vi "Create.vi"(10 "Groups":string[](array[string])) -> (3 "GroupsValue out":refnum<class "GroupsValue.lvclass">)   [LabVIEW 2020, in "Vecto.lvlib" / "GroupsValue.lvclass"]
uses:
  GroupsValue.lvclass
  GroupsValue.lvclass/GroupsValue.ctl
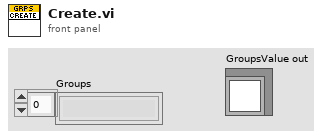
[diagram p1: front panel]
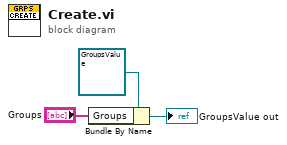
[diagram p0: block diagram]
diagram:
  n1 = Bundle By Name(cluster=refnum<class "GroupsValue.lvclass"> refnum ("GroupsValue out"), "Groups"="Groups") -> (→"GroupsValue out":refnum<class "GroupsValue.lvclass">)
